vi "Animation - AVI.vi"() -> ()   [LabVIEW 2013]
doc: "Sample numeric display item."
uses:
  <vilib>/NI Veristand/Display Template Support/Display Template Support.llb/cluster_Screen Item Settings.ctl
  <vilib>/NI Veristand/Display Template Support/Display Template Support.llb/cluster_Graph Scale Settings.ctl
  <vilib>/NI Veristand/Display Template Support/Display Template Support.llb/cluster_Graph Plot Settings.ctl
  <vilib>/NI Veristand/Display Template Support/Display Template Support.llb/enum_Display Template Handler Minimal To Widget Msg.ctl
  <vilib>/NI Veristand/Display Template Support/Display Template Support.llb/enum_Display Template Handler Minimal To Workspace.ctl
  <vilib>/NI Veristand/Execution/Workspace/SystemStateRegEventRef.ctl
  <vilib>/NI Veristand/Execution/Workspace/WorkspaceAPI.ctl
  <vilib>/NI Veristand/Execution/Workspace/SystemStateEventRef.ctl
  Supporting Files/Animation Cluster.ctl
  <vilib>/vision/Avi1.llb/AviRefnum.ctl
  <vilib>/vision/Image Controls.llb/IMAQ Image.ctl
  <vilib>/NI Veristand/Execution/Workspace/SystemState.ctl
  <vilib>/NI Veristand/Display Template Support/Display Template Support.llb/sub_Display Template Handler Custom.vi
  <userlib>/QMH/QMH Add Message to Queue (Single Element).vi
  <userlib>/QMH/QMH Add Message to Queue (Array).vi
  <vilib>/NI Veristand/Execution/Workspace/NI_VS Workspace ExecutionAPI.lvlib
  NationalInstruments.VeriStand.ClientAPI
panel:
  out "Image":T1(plugin-control)
  in  "NIVS.Gateway IP Address":string
  in  "Item.Data":T2
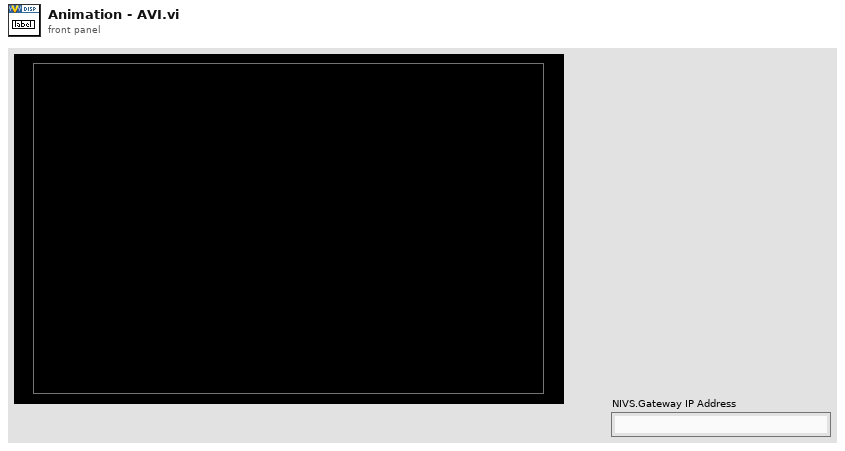
[diagram p1: front panel]
types:
  T1 = typedef "IMAQ Image.ctl" = refnum<image>
  T2 = typedef "cluster_Screen Item Settings.ctl" = cluster{"Template VI":string, "Position X":i32, "Position Y":i32, "Custom":string, "Show Title Bar":bool, "ID":i32, "Always On Top":bool, "Allow Resize":bool, "Allow Minimize":bool, "Allow Close":bool, "Size to Screen":bool, "Screen.ID":i32, "State":enum16{"Normal", "New"}, "Title":string, "Window Bounds":cluster{"[0]":i16, "[1]":i16, "[2]":i16, "[3]":i16}, "Channel Ref":u64, "Unit":string, "Default Units?":bool, "Flash Limit?":bool, "Color 1":u32, "Color 2":u32, "Color 3":u32, "Color 4":u32, "Bck Color":u32, "Fore Color":u32, "Limit 1":dbl, "Limit 2":dbl, "Limit 3":dbl, "Limit 4":dbl, "Limit Mode 1":i32, "Limit Mode 2":i32, "Limit Mode 3":i32, "Limit Mode 4":i32, "Scale Precision":i32, "Scale Min":dbl, "Scale Max":dbl, "Format":i32, "Precision":i32, "Background Type":i32, "IDs":i32[], "Units":string[], "Labels":string[], "Scale Factor":dbl, "Scale Offset":dbl, "YScale Index":u32[], "XScale":T3, "YScales":T3[], "Plots":T4[], "Update Period":dbl, "History Length":dbl, "My.Ref":refnum<vi>, "Is Control?":bool, "Channel Paths":string[], "Custom Data":variant}
  T3 = typedef "cluster_Graph Scale Settings.ctl" = cluster{"Format":u8, "Precision":u8, "Fit":u8, "Label":string, "Use Default Label":bool, "Label Visible":bool, "Min":dbl, "Max":dbl}
  T4 = typedef "cluster_Graph Plot Settings.ctl" = cluster{"Bar Style":u8, "Fill To":i16, "Fill/PtColor":u32, "Line Style":u8, "Line Width":u8, "Color":u32, "Interp":u8, "Point Style":u8}
  T5 = typedef "Animation Cluster.ctl" = cluster{"AVI path":path, "Frame Number":u32}
  T6 = typedef "enum_Display Template Handler Minimal To Workspace.ctl" = cluster{"Operation":enum16{"SetCustomData", "DeleteItem"}, "Data":variant}
  T7 = typedef "enum_Display Template Handler Minimal To Widget Msg.ctl" = enum16{"Stop", "LaunchConfigDialog"}
  T8 = typedef "NI_VS Workspace ExecutionAPI.lvlib/SystemStateRegEventRef.ctl" = refnum<event-registration>
  T9 = typedef "NI_VS Workspace ExecutionAPI.lvlib/WorkspaceAPI.ctl" = refnum<k24>
  T10 = typedef "NI_VS Workspace ExecutionAPI.lvlib/SystemStateEventRef.ctl" = cluster{"CustDatRef":refnum<user-event>, "EvtRef":refnum<k27>}
  T11 = typedef "AviRefnum.ctl" = refnum<k1>
  T12 = cluster{"LaunchConfigDialog":refnum<user-event>, "Set Custom Data":refnum<user-event>, "Registered Events":cluster{"Event Registration Refnum":refnum<event-registration>, "SystemChangeEventRef":T8}, "WorkspaceManager Ref":T9, "SystemStateRefs":T10, "Custom Data":T5, "Avi Refnum":T11, "Image Name":string, "ms per frame":i32, "Number of Frames":u32, "Image Ref":T1, "Play":bool}
  T13 = cluster{"Event Registration Refnum":refnum<event-registration>, "SystemChangeEventRef":T8}
  T14 = typedef "NI_VS Workspace ExecutionAPI.lvlib/SystemState.ctl" = u8
  T15 = typedef "Image Type" = u32
  T16 = cluster{"width":u32, "height":u32, "framesPerSecond":u32, "compressionFilter":string, "hasData":bool}
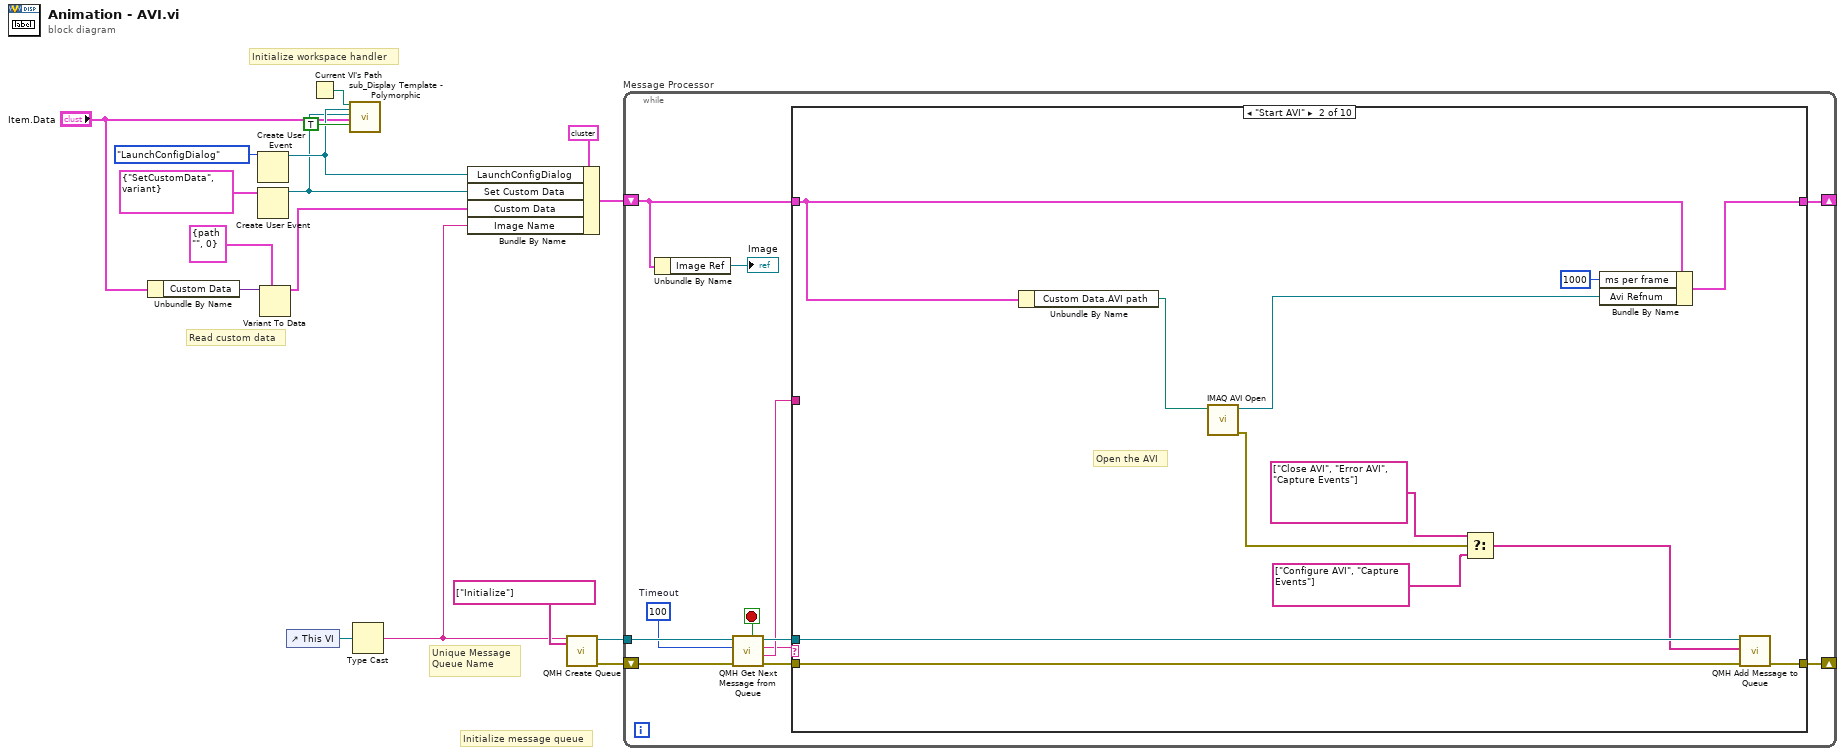
[diagram p0: block diagram]
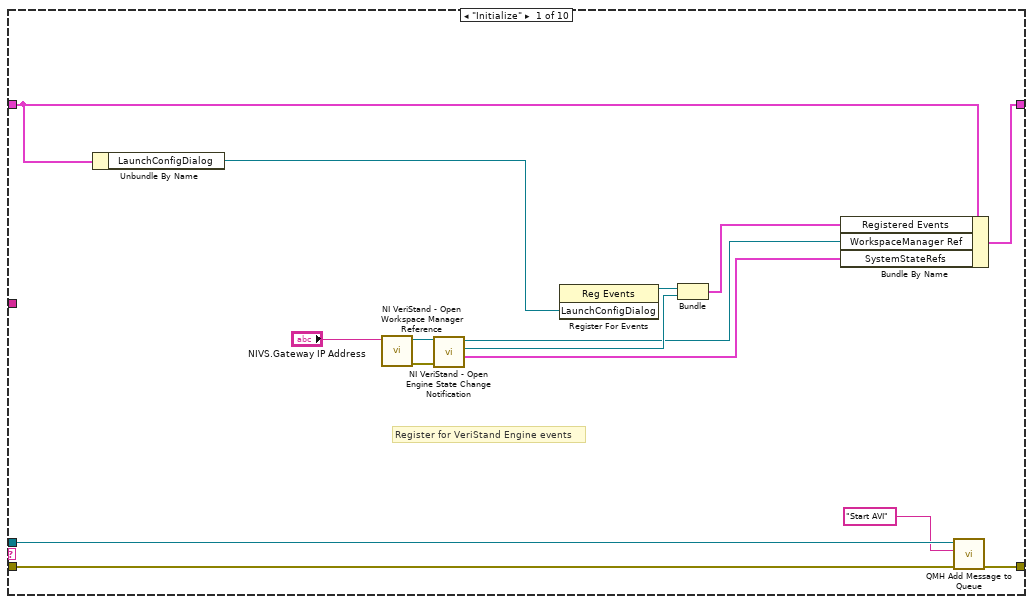
[diagram p2: hidden frame]
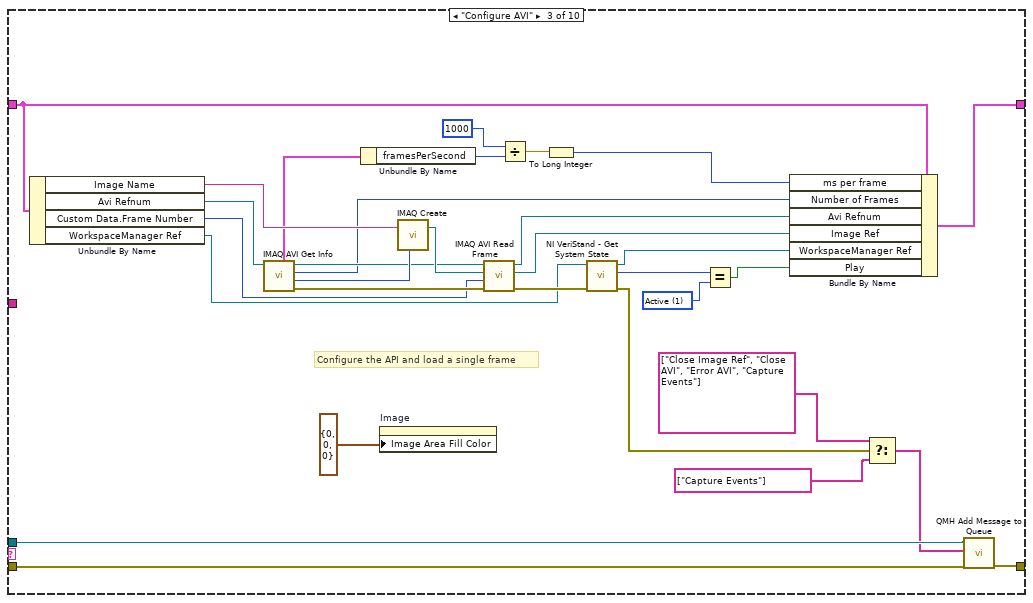
[diagram p3: hidden frame]
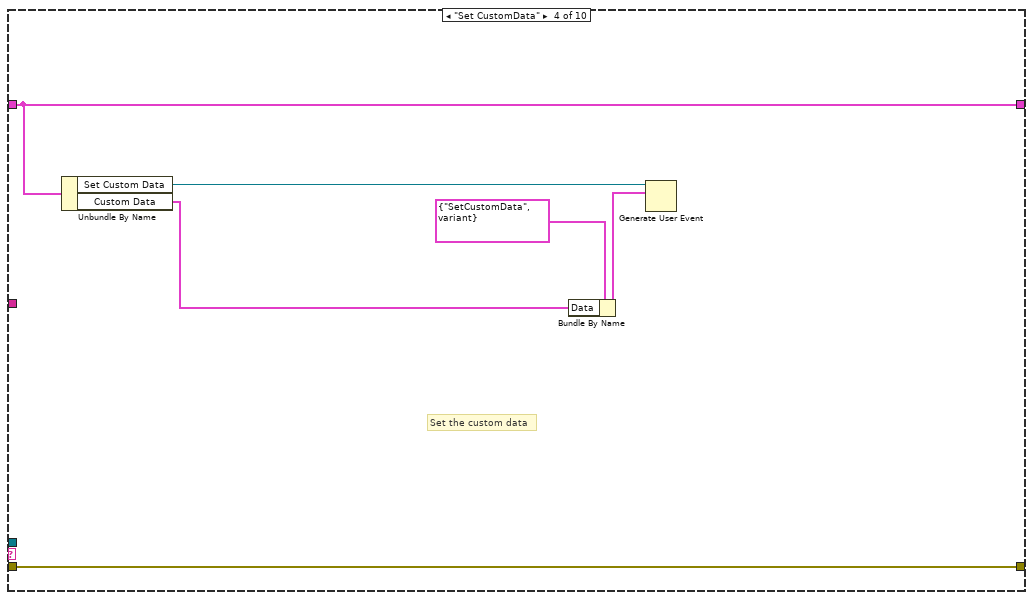
[diagram p4: hidden frame]
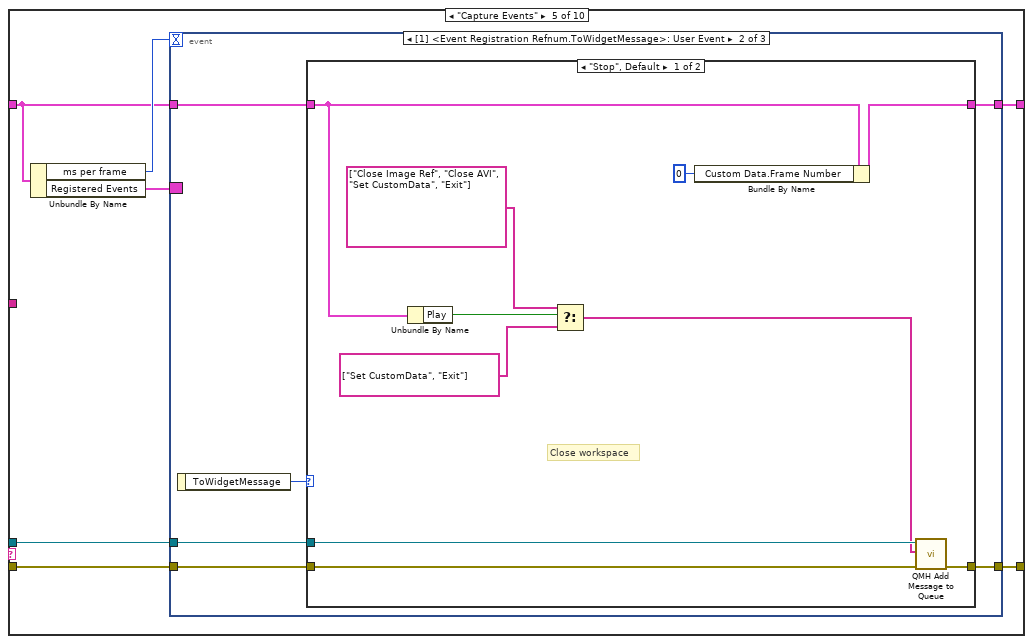
[diagram p5: hidden frame]
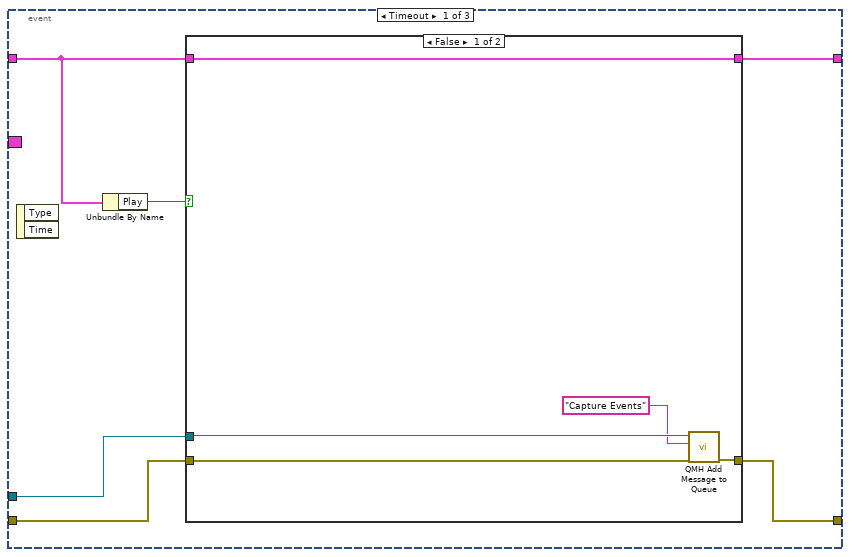
[diagram p6: hidden frame]
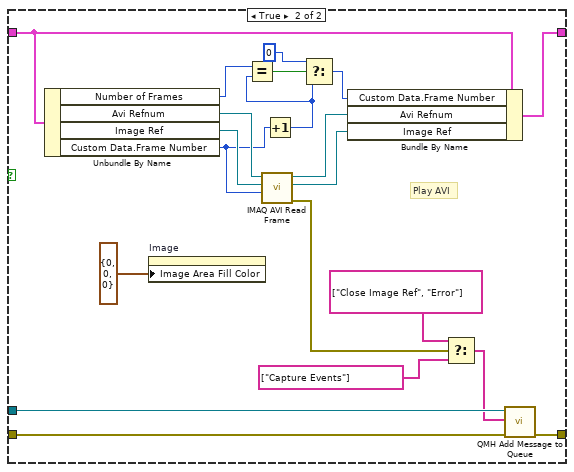
[diagram p7: hidden frame]
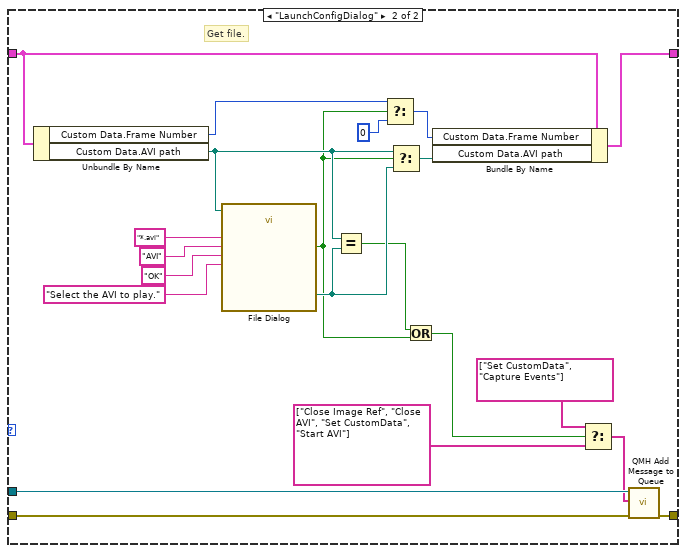
[diagram p8: hidden frame]
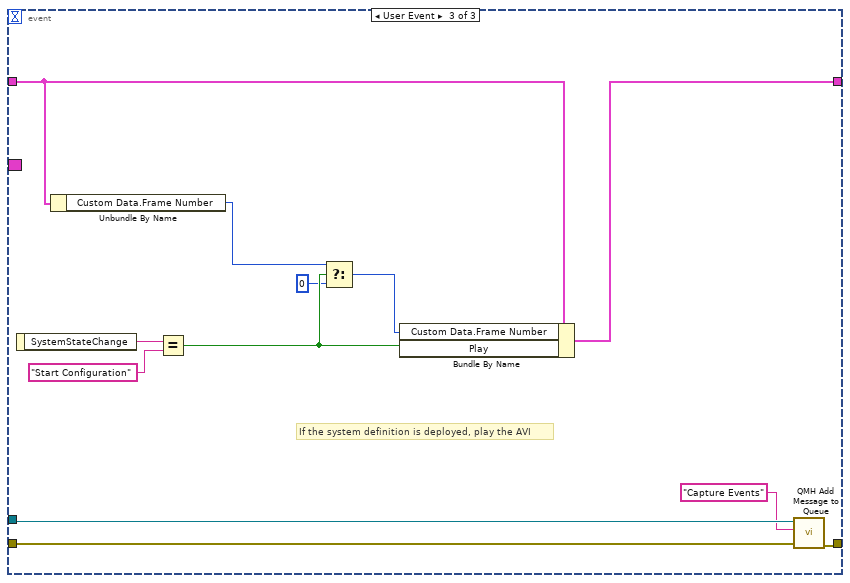
[diagram p9: hidden frame]
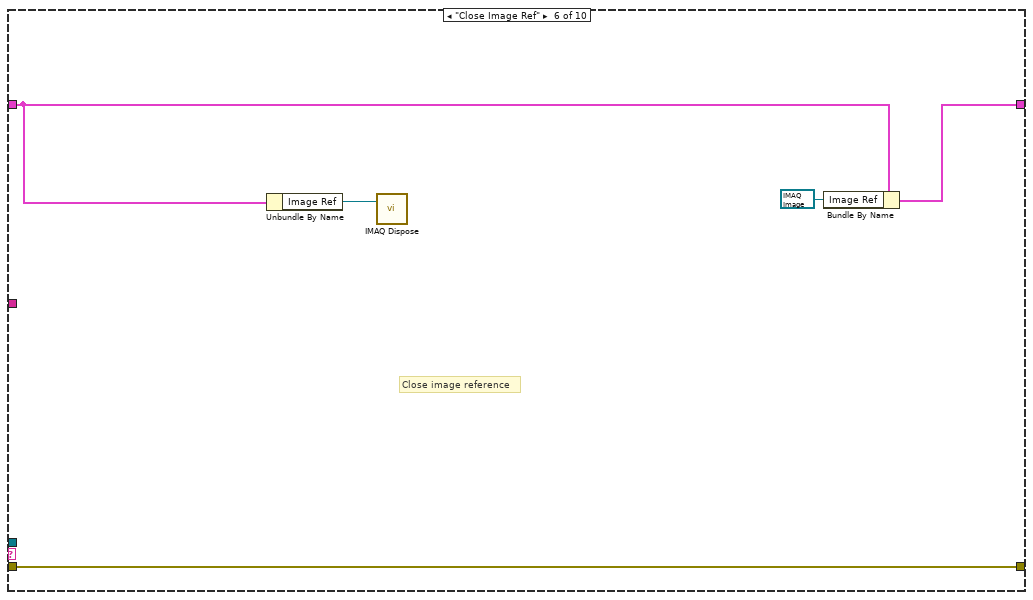
[diagram p10: hidden frame]
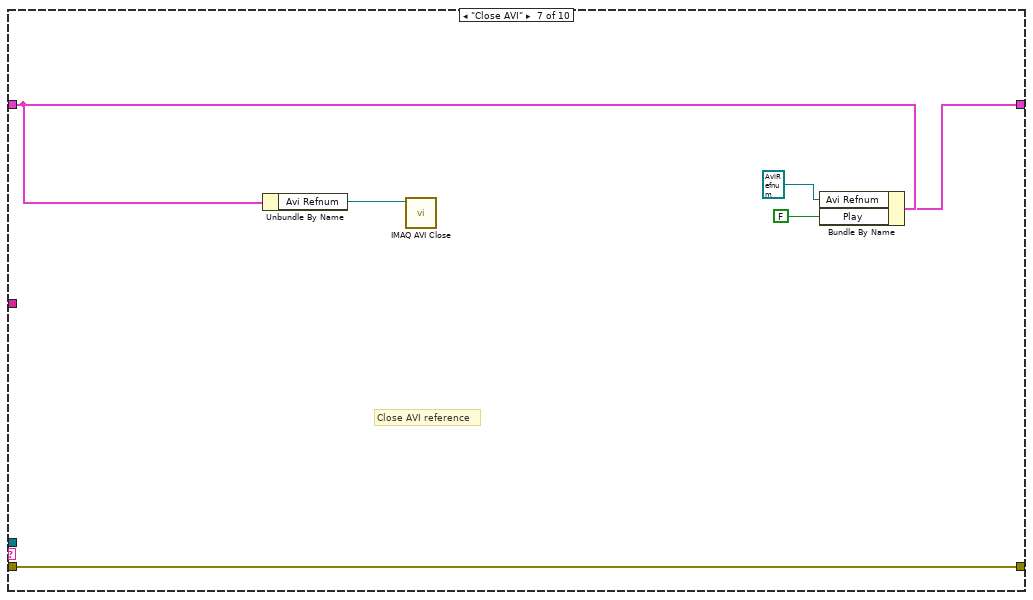
[diagram p11: hidden frame]
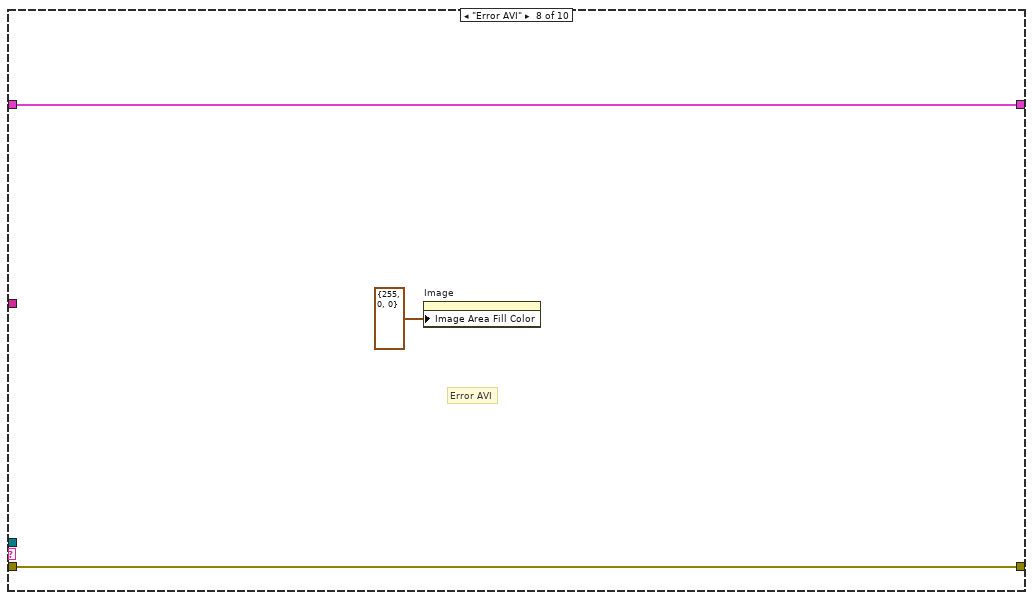
[diagram p12: hidden frame]
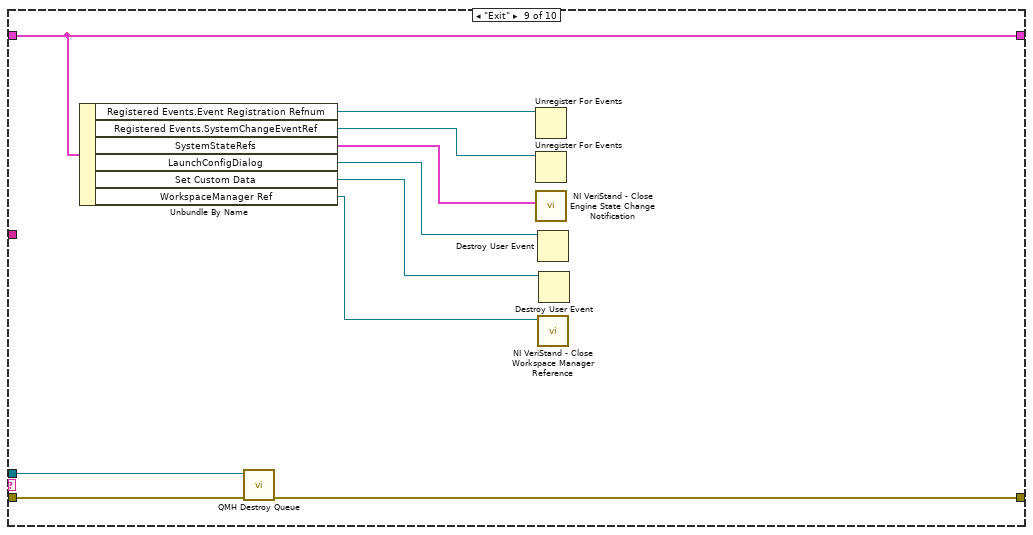
[diagram p13: hidden frame]
diagram:
  # "Read custom data"
  # "Initialize workspace handler"
  # "Initialize message queue"
  # "Unique Message\nQueue Name"
  n1 = Unbundle By Name("Item.Data") -> ("Custom Data"=w3:variant)
  n2 = Create User Event(user event datatype=enum_Display_Template_Handler_Minimal_To_Widget_Msg."LaunchConfigDialog" ("ToWidgetMessage")) -> (user event=w7:refnum<user-event>)  [unwired: 1 in, 1 out]
  n3 = Create User Event(user event datatype=T6 {"Operation"=enum."SetCustomData", "Data"=variant} ("Data")) -> (user event=w6:refnum<user-event>)  [unwired: 1 in, 1 out]
  n4 = Variant To Data(type=T5 {"AVI path"=path "", "Frame Number"=0} ("Animation Cluster"), Variant=w3) -> (data=w1:T5)  [unwired: 1 in, 1 out]
  n5 = control-ref of="This VI"() -> (w14:refnum<vi>)
  n6 = Current VI's Path() -> (path=w9:path)
  n7 = call-poly <vilib>:"sub_Display Template - Polymorphic.vi"("Parent.Path"=w9, "ToWidgetEvent"=w7, "ToWorkspace"=w6, "Item.Data"="Item.Data", "Resizable"=TRUE) -> ()  [unwired: 1 in, 14 out]
  n8 = Type Cast(x=w14) -> (*(type *) &x=w5:string)  [unwired: 1 in]
  n9 = Bundle By Name(cluster=T12 {"LaunchConfigDialog"=refnum, "Set Custom Data"=refnum, "Registered Events"={"Event Registration Refnum"=refnum, "SystemChangeEventRef"=refnum}, "WorkspaceManager Ref"=refnum, "SystemStateRefs"={"CustDatRef"=refnum, "EvtRef"=refnum}, "Custom Data"={"AVI path"=path "", "Frame Number"=0}, "Avi Refnum"=refnum, "Image Name"="untitled", "ms per frame"=0, "Number of Frames"=0, "Image Ref"=refnum, "Play"=FALSE}, "LaunchConfigDialog"=w7, "Set Custom Data"=w6, "Custom Data"=w1, "Image Name"=w5) -> (w12:T12)
  n10 = call <userlib>:"QMH Create Queue.vi"("Initial Messages"=string[] ["Initialize"], "Message queue name (unnamed)"=w5) -> ("error out"=w15:errorcluster, "queue out"=w16:refnum<queue>)  [unwired: 8 in]
  n11 = while "Message Processor" {
    shift-left: w15 -> [w25]
    shift-right: [w29] -> _
    tunnel: w16 -> [w26]
    shift-right: [w21] -> _
    shift-left: w12 -> [w19]
    stop <- w28 stop-if-true
    w23 = 100  # Timeout
    n12 = Unbundle By Name(w19) -> ("Image Ref"=→"Image":T1)
    n13 = call <userlib>:"QMH Get Next Message from Queue.vi"("error in (no error)"=w25, "ms timeout (1)"=w23, "queue in"=w26) -> ("error out"=w24:errorcluster, "Next Parameter"=w22:string, "Next Message"=w20:string, "queue out"=w27:refnum<queue>, "Stop QMH"=w28:bool)  [unwired: 3 in]
    n14 = case shown="\"Start AVI\"" w20 {
      tunnel: w27 -> [w34 w50 w70 _ w96 _ _ _ w203 _]
      tunnel: w24 -> [w32 w45 w66 w93 w94 w183 w187 w194 w204 w205]
      tunnel: [w35 w51 w71 w93 w97 w183 w187 w194 w202 w205] -> w29
      tunnel: w22 -> [_ _ _ _ _ _ _ _ _ _]
      tunnel: w19 -> [w31 w55 w87 w92 w98 w185 w191 w192 w201 w206]
      tunnel: [w39 w53 w86 w92 w95 w184 w190 w192 w201 w206] -> w21
      frame "Initialize" {
        # "Register for VeriStand Engine events"
        n15 = Unbundle By Name(w31) -> ("LaunchConfigDialog"=w30:refnum<user-event>)
        n16 = call <vilib>:"NI VeriStand - Open Workspace Manager Reference.vi"("Gateway IP Address (\"\": localhost)"="NIVS.Gateway IP Address") -> ("error out"=w44:errorcluster, "WorkspaceManager"=w43:T9)  [unwired: 9 in]
        n17 = call <vilib>:"NI VeriStand - Open Engine State Change Notification.vi"("error in (no error)"=w44, "WorkspaceManager in"=w43) -> ("SystemStateRefs"=w36:T10, "SystemChangeEventRef"=w40:T8, "WorkspaceManager out"=w37:T9)  [unwired: 6 in, 1 out]
        n18 = register-events(w30) -> (reference out=w41:refnum<event-registration>)  [unwired: 2 in, 1 out]
        n19 = Bundle("Event Registration Refnum"=w41, "SystemChangeEventRef"=w40) -> (w38:T13)  [unwired: 1 in]
        n20 = Bundle By Name(cluster=w31, "Registered Events"=w38, "WorkspaceManager Ref"=w37, "SystemStateRefs"=w36) -> (w39:T12)
        n21 = call-poly <userlib>:"QMH Add Message to Queue.vi"("error in (no error)"=w32, "Message"="Start AVI" ("Message Name"), "queue in"=w34) -> ("error out"=w35:errorcluster)  [unwired: 7 in, 1 out]
      }
      frame "Start AVI" {
        # "Open the AVI"
        n22 = Unbundle By Name(w55) -> ("Custom Data.AVI path"=w56:path)
        n23 = call "IMAQ AVI Open"("AVI Path"=w56) -> ("error out"=w52:errorcluster, "Avi Refnum"=w54:T11)  [unwired: 9 in]
        n24 = Select(t=string[] ["Close AVI", "Error AVI", "Capture Events"] ("Message Names"), s=w52, f=string[] ["Configure AVI", "Capture Events"] ("Message Names")) -> (s? t:f=w47:string[])
        n25 = Bundle By Name(cluster=w55, "ms per frame"=1000, "Avi Refnum"=w54) -> (w53:T12)
        n26 = call-poly <userlib>:"QMH Add Message to Queue.vi"("error in (no error)"=w45, "Messages"=w47, "queue in"=w50) -> ("error out"=w51:errorcluster)  [unwired: 7 in, 1 out]
      }
      frame "Configure AVI" {
        w60 = T14 1 items=["Idle", "Active"] ("y")
        # "Configure the API and load a single frame"
        n27 = Unbundle By Name(w87) -> ("Image Name"=w82:string, "Avi Refnum"=w85:T11, "Custom Data.Frame Number"=w79:u32, "WorkspaceManager Ref"=w64:T9)
        n28 = call "IMAQ AVI Get Info"("Avi Refnum"=w85) -> ("error out"=w84:errorcluster, "Image Type"=w83:T15, "Number of Frames"=w73:u32, "Avi Refnum (duplicate)"=w80:T11, "Frame Data"=w78:T16)  [unwired: 6 in]
        n29 = Unbundle By Name(w78) -> ("framesPerSecond"=w77:u32)
        n30 = property on="Image" class="ImageControl"("Image Area Fill Color"=cluster{"Red":u8, "Green":u8, "Blue":u8} {"Red"=0, "Green"=0, "Blue"=0} ("Image Area:Background:Fill Color")) -> ()  [unwired: 2 in, 2 out]
        n31 = call "IMAQ Create"("Image Name"=w82, "Image Type"=w83) -> ("New Image"=w81:T1)  [unwired: 3 in, 1 out]
        n32 = call "IMAQ AVI Read Frame"("error in (no error)"=w84, "Frame Number"=w79, "Image"=w81, "Avi Refnum"=w80) -> ("error out"=w65:errorcluster, "Image Out"=w58:T1, "Avi Refnum (duplicate)"=w72:T11)  [unwired: 4 in, 1 out]
        n33 = Divide(x=u32 1000, y=w77) -> (x/y=w75:dbl)
        n34 = To Long Integer(number=w75) -> (32bit integer=w74:i32)
        n35 = call <vilib>:"NI VeriStand - Get System State.vi"("error in (no error)"=w65, "WorkspaceManager in"=w64) -> ("error out"=w62:errorcluster, "System State"=w61:T14, "WorkspaceManager  out"=w63:T9)  [unwired: 5 in, 2 out]
        n36 = Equal?(x=w61, y=w60) -> (x = y?=w59:bool)
        n37 = Bundle By Name(cluster=w87, "ms per frame"=w74, "Number of Frames"=w73, "Avi Refnum"=w72, "Image Ref"=w58, "WorkspaceManager Ref"=w63, "Play"=w59) -> (w86:T12)
        n38 = Select(t=string[] ["Close Image Ref", "Close AVI", "Error AVI", "Capture Events"] ("Message Names"), s=w62, f=string[] ["Capture Events"] ("Message Names")) -> (s? t:f=w67:string[])
        n39 = call-poly <userlib>:"QMH Add Message to Queue.vi"("error in (no error)"=w66, "Messages"=w67, "queue in"=w70) -> ("error out"=w71:errorcluster)  [unwired: 7 in, 1 out]
      }
      frame "Set CustomData" {
        # "Set the custom data"
        n40 = Unbundle By Name(w92) -> ("Set Custom Data"=w89:refnum<user-event>, "Custom Data"=w88:T5)
        n41 = Bundle By Name(cluster=T6 {"Operation"=enum."SetCustomData", "Data"=variant} ("event data"), "Data"=w88) -> (w90:T6)
        n42 = Generate User Event(user event=w89, event data cluster=w90) -> ()  [unwired: 2 in, 2 out]
      }
      frame "Capture Events" {
        n43 = Unbundle By Name(w98) -> ("ms per frame"=w99:i32, "Registered Events"=w100:T13)
        n44 = event shown="[1] <Event Registration Refnum.ToWidgetMessage>: User Event" {
          selector: w100 -> [_ _ _]
          dyn-events: _ -> [_ _ _]
          timeout: w99 -> [_ _ _]
          tunnel: w98 -> [w105 w136 w173]
          tunnel: [w101 w135 w177] -> w97
          tunnel: w96 -> [w103 w134 w175]
          tunnel: [w104 w133 w178] -> w95
          tunnel: w94 -> [w102 w132 w176]
          event Timeout {
            n45 = event-data() -> ()  [unwired: 1 in, 2 out]
            n46 = Unbundle By Name(w105) -> ("Play"=w106:bool)
            n47 = case shown="False" w106 {
              tunnel: w105 -> [w111 w129]
              tunnel: [w111 w127] -> w104
              tunnel: w103 -> [w109 w125]
              tunnel: w102 -> [w108 w124]
              tunnel: [w110 w123] -> w101
              frame False {
                n48 = call-poly <userlib>:"QMH Add Message to Queue.vi"("error in (no error)"=w108, "Message"="Capture Events" ("Message Name"), "queue in"=w109) -> ("error out"=w110:errorcluster)  [unwired: 7 in, 1 out]
              }
              frame True {
                # "Play AVI"
                n49 = Unbundle By Name(w129) -> ("Number of Frames"=w116:u32, "Avi Refnum"=w131:T11, "Image Ref"=w130:T1, "Custom Data.Frame Number"=w115:u32)
                n50 = property on="Image" class="ImageControl"("Image Area Fill Color"=cluster{"Red":u8, "Green":u8, "Blue":u8} {"Red"=0, "Green"=0, "Blue"=0} ("Image Area:Background:Fill Color")) -> ()  [unwired: 2 in, 2 out]
                n51 = call "IMAQ AVI Read Frame"("Frame Number"=w115, "Image"=w130, "Avi Refnum"=w131) -> ("error out"=w121:errorcluster, "Image Out"=w126:T1, "Avi Refnum (duplicate)"=w128:T11)  [unwired: 5 in, 1 out]
                n52 = Increment(x=w115) -> (x+1=w113:u32)
                n53 = Equal?(x=w116, y=w113) -> (x = y?=w118:bool)
                n54 = Select(t=u32 0 ("Number of Frames"), s=w118, f=w113) -> (s? t:f=w114:u32)
                n55 = Bundle By Name(cluster=w129, "Custom Data.Frame Number"=w114, "Avi Refnum"=w128, "Image Ref"=w126) -> (w127:T12)
                n56 = Select(t=string[] ["Close Image Ref", "Error"] ("Message Names"), s=w121, f=string[] ["Capture Events"]) -> (s? t:f=w120:string[])
                n57 = call-poly <userlib>:"QMH Add Message to Queue.vi"("error in (no error)"=w124, "Messages"=w120, "queue in"=w125) -> ("error out"=w123:errorcluster)  [unwired: 7 in, 1 out]
              }
            }
          }
          event User Event {
            n58 = event-data() -> ("ToWidgetMessage"=w137:T7)  [unwired: 1 in]
            n59 = case shown="\"Stop\", Default" w137 {
              tunnel: w136 -> [w140 w162]
              tunnel: [w146 w164] -> w135
              tunnel: w134 -> [w145 w163]
              tunnel: [w139 w160] -> w133
              tunnel: w132 -> [w147 w156]
              frame "Stop", Default {
                # "Close workspace"
                n60 = Unbundle By Name(w140) -> ("Play"=w144:bool)
                n61 = Select(t=string[] ["Close Image Ref", "Close AVI", "Set CustomData", "Exit"] ("Message Names"), s=w144, f=string[] ["Set CustomData", "Exit"] ("Message Names")) -> (s? t:f=w142:string[])
                n62 = Bundle By Name(cluster=w140, "Custom Data.Frame Number"=u32 0) -> (w139:T12)
                n63 = call-poly <userlib>:"QMH Add Message to Queue.vi"("error in (no error)"=w147, "Messages"=w142, "queue in"=w145) -> ("error out"=w146:errorcluster)  [unwired: 7 in, 1 out]
              }
              frame "LaunchConfigDialog" {
                # "Get file."
                n64 = Unbundle By Name(w162) -> ("Custom Data.Frame Number"=w158:u32, "Custom Data.AVI path"=w152:path)
                n65 = call "File Dialog"("start path"=w152, "prompt"="Select the AVI to play.", "button label"="OK", "pattern (all files)"="*.avi", "pattern label"="AVI") -> ("selected path"=w151:path, "cancelled"=w150:bool)  [unwired: 7 in, 2 out]
                n66 = Equal?(x=w152, y=w151) -> (x = y?=w149:bool)
                n67 = Select(t=w158, s=w150, f=u32 0) -> (s? t:f=w159:u32)
                n68 = Select(t=w152, s=w150, f=w151) -> (s? t:f=w161:path)
                n69 = Or(x=w149, y=w150) -> (x .or. y?=w148:bool)
                n70 = Bundle By Name(cluster=w162, "Custom Data.Frame Number"=w159, "Custom Data.AVI path"=w161) -> (w160:T12)
                n71 = Select(t=string[] ["Set CustomData", "Capture Events"] ("Message Names"), s=w148, f=string[] ["Close Image Ref", "Close AVI", "Set CustomData", "Start AVI"] ("Message Names")) -> (s? t:f=w153:string[])
                n72 = call-poly <userlib>:"QMH Add Message to Queue.vi"("error in (no error)"=w156, "Messages"=w153, "queue in"=w163) -> ("error out"=w164:errorcluster)  [unwired: 7 in, 1 out]
              }
            }
          }
          event User Event {
            # "If the system definition is deployed, play the AVI"
            n73 = event-data() -> ("SystemStateChange"=w180:string)  [unwired: 1 in]
            n74 = Unbundle By Name(w173) -> ("Custom Data.Frame Number"=w171:u32)
            n75 = Equal?(x=w180, y="Start Configuration") -> (x = y?=w172:bool)
            n76 = Select(t=w171, s=w172, f=u32 0) -> (s? t:f=w170:u32)
            n77 = Bundle By Name(cluster=w173, "Custom Data.Frame Number"=w170, "Play"=w172) -> (w178:T12)
            n78 = call-poly <userlib>:"QMH Add Message to Queue.vi"("error in (no error)"=w176, "Message"="Capture Events" ("Message Name"), "queue in"=w175) -> ("error out"=w177:errorcluster)  [unwired: 7 in, 1 out]
          }
        }
      }
      frame "Close Image Ref" {
        # "Close image reference"
        n79 = Unbundle By Name(w185) -> ("Image Ref"=w182:T1)
        n80 = call "IMAQ Dispose"("Image"=w182) -> ()  [unwired: 5 in, 1 out]
        n81 = Bundle By Name(cluster=w185, "Image Ref"=T1 refnum) -> (w184:T12)
      }
      frame "Close AVI" {
        # "Close AVI reference"
        n82 = Unbundle By Name(w191) -> ("Avi Refnum"=w188:T11)
        n83 = call "IMAQ AVI Close"("Avi Refnum"=w188) -> ()  [unwired: 10 in, 1 out]
        n84 = Bundle By Name(cluster=w191, "Avi Refnum"=T11 refnum, "Play"=FALSE) -> (w190:T12)
      }
      frame "Error AVI" {
        # "Error AVI"
        n85 = property on="Image" class="ImageControl"("Image Area Fill Color"=cluster{"Red":u8, "Green":u8, "Blue":u8} {"Red"=255, "Green"=0, "Blue"=0} ("Image Area:Background:Fill Color")) -> ()  [unwired: 2 in, 2 out]
      }
      frame "Exit" {
        n86 = Unbundle By Name(w201) -> ("Registered Events.Event Registration Refnum"=w200:refnum<event-registration>, "Registered Events.SystemChangeEventRef"=w199:T8, "SystemStateRefs"=w198:T10, "LaunchConfigDialog"=w197:refnum<user-event>, "Set Custom Data"=w196:refnum<user-event>, "WorkspaceManager Ref"=w195:T9)
        n87 = call <userlib>:"QMH Destroy Queue.vi"("error in (no error)"=w204, "queue in"=w203) -> ("error out"=w202:errorcluster)  [unwired: 7 in, 2 out]
        n88 = Unregister For Events(event registration refnum=w200) -> ()  [unwired: 1 in, 1 out]
        n89 = Unregister For Events(event registration refnum=w199) -> ()  [unwired: 1 in, 1 out]
        n90 = call <vilib>:"NI VeriStand - Close Engine State Change Notification.vi"("SystemStateRefs"=w198) -> ()  [unwired: 10 in, 1 out]
        n91 = Destroy User Event(user event=w197) -> ()  [unwired: 1 in, 1 out]
        n92 = call <vilib>:"NI VeriStand - Close Workspace Manager Reference.vi"("WorkspaceManager"=w195) -> ()  [unwired: 10 in, 1 out]
        n93 = Destroy User Event(user event=w196) -> ()  [unwired: 1 in, 1 out]
      }
      frame Default {
      }
    }
  }
